vi "_builtins_resize_window.vi"(8 "error in (no error)":errorcluster, 10 "Focus":enum8{"FP", "BD"}(ring), 11 "VI Refnum in":refnum<vi>) -> (0 "error out":errorcluster, 3 "VI Refnum out":refnum<vi>)   [LabVIEW 2019, in "Script.lvlib"]
doc: "Resizes the front panel or block diagram window to content. On the front panel, this also resets the origins to 0, 0.\n\nCreated by: Ryan Pacini"
uses:
  Script.lvlib
  <vilib>/Utility/miscctls.llb/LVBoundsTypeDef.ctl
  <vilib>/Utility/miscctls.llb/LVPointTypeDef.ctl
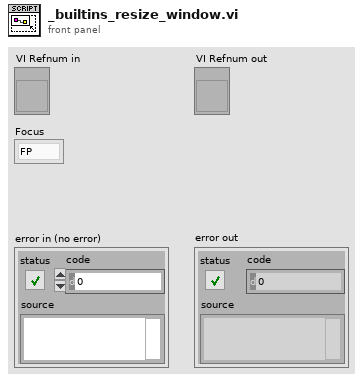
[diagram p1: front panel]
types:
  T1 = typedef "LVAllMonitorsDisplayTypeDef.ctl" = cluster{"Bounds":cluster{"Left":i16, "Top":i16, "Right":i16, "Bottom":i16}, "Depth":i16}[]
  T2 = typedef "LVBoundsTypeDef.ctl" = cluster{"Width":u32, "Height":u32}
  T3 = cluster{"Left":i16, "Top":i16, "Right":i16, "Bottom":i16}
  T4 = typedef "LVRectTypeDef.ctl" = cluster{"Left":i16, "Top":i16, "Right":i16, "Bottom":i16}
  T5 = typedef "LVPointTypeDef.ctl" = cluster{"Horizontal":i16, "Vertical":i16}
  T6 = typedef "LVPositionTypeDef.ctl" = cluster{"Left":i32, "Top":i32}
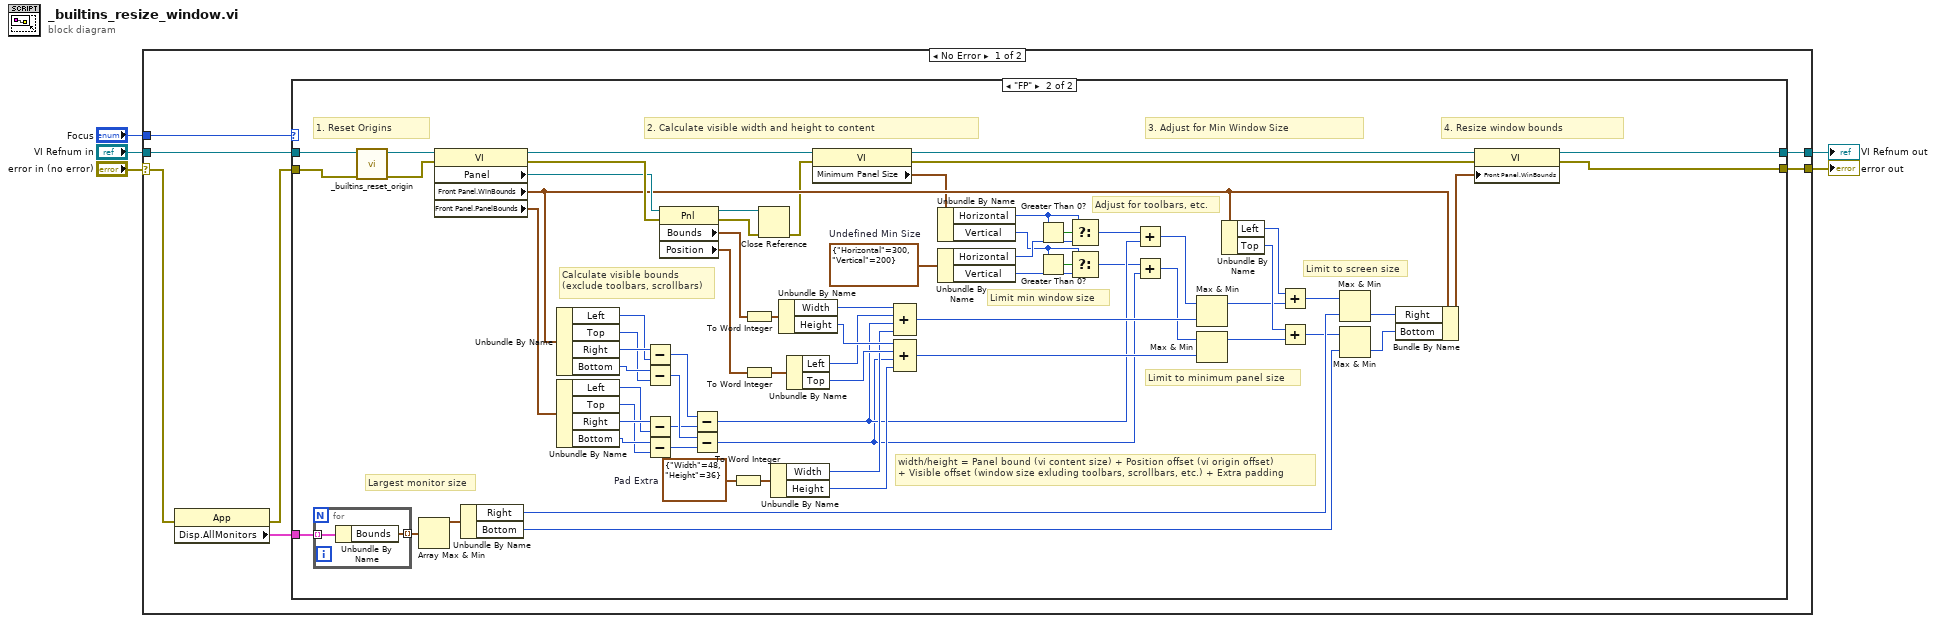
[diagram p0: block diagram]
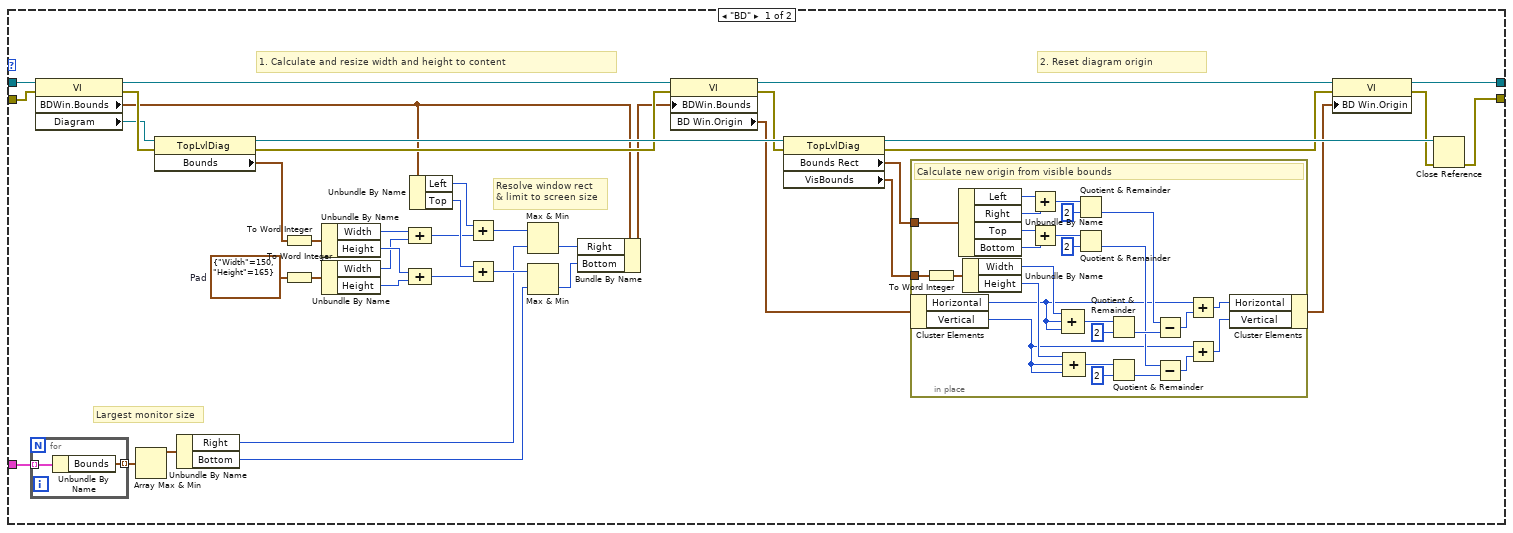
[diagram p2: hidden frame]
diagram:
  n1 = case shown="No Error" "error in (no error)" {
    selector: "error in (no error)" -> [w7 w155]
    tunnel: [w12 w156] -> w5
    tunnel: "VI Refnum in" -> [w11 w156]
    tunnel: [w10 w155] -> w2
    tunnel: "Focus" -> [w9 _]
    frame No Error {
      n2 = property class="App"(error in=w7) -> (error out=w6:errorcluster, "Disp.AllMonitors"=w8:T1)  [unwired: 1 in, 1 out]
      n3 = case shown="\"FP\"" w9 {
        tunnel: [w53 w152] -> w12
        tunnel: w11 -> [w52 w109]
        tunnel: w6 -> [w51 w111]
        tunnel: [w36 w107] -> w10
        tunnel: w8 -> [w14 w113]
        frame "BD" {
          w17 = T2 {"Width"=150, "Height"=165}  # Pad
          # "Largest monitor size"
          # "2. Reset diagram origin"
          # "1. Calculate and resize width and height to content"
          # "Resolve window rect\n& limit to screen size"
          n4 = for {
            tunnel: w14 -> [w82] mode=indexing
            tunnel: [w81] -> w37 mode=indexing
            n5 = Unbundle By Name(w82) -> ("Bounds"=w81:T3)
          }
          n6 = property on="Property Node" class="VI"(reference=w52, error in=w51) -> (reference out=w13:refnum<vi>, error out=w43:errorcluster, "BDWin.Bounds"=w25:T4, "Diagram"=w19:refnum<vi>)
          n7 = Array Max & Min(array=w37) -> (max value=w44:T3)  [unwired: 3 out]
          n8 = property on="Property Node" class="TopLvlDiag"(reference=w19, error in=w43) -> (reference out=w49:refnum<vi>, error out=w42:errorcluster, "Bounds"=w34:T2)
          n9 = Unbundle By Name(w44) -> ("Right"=w22:i16, "Bottom"=w21:i16)
          n10 = To Word Integer(number=w34) -> (16bit integer=w35:cluster{"Width":i16, "Height":i16})
          n11 = To Word Integer(number=w17) -> (16bit integer=w18:cluster{"Width":i16, "Height":i16})
          n12 = Unbundle By Name(w35) -> ("Width"=w32:i16, "Height"=w33:i16)
          n13 = Unbundle By Name(w18) -> ("Width"=w15:i16, "Height"=w16:i16)
          n14 = Compound Arithmetic op=ADD(w32, w15) -> (w24:i16)
          n15 = Compound Arithmetic op=ADD(w33, w16) -> (w23:i16)
          n16 = Unbundle By Name(w25) -> ("Left"=w29:i16, "Top"=w26:i16)
          n17 = Add(x=w29, y=w24) -> (x+y=w28:i16)
          n18 = Add(x=w26, y=w23) -> (x+y=w27:i16)
          n19 = Max & Min(x=w28, y=w22) -> (min(x,y)=w30:i16)  [unwired: 1 out]
          n20 = Max & Min(x=w27, y=w21) -> (min(x,y)=w31:i16)  [unwired: 1 out]
          n21 = Bundle By Name(cluster=w25, "Right"=w30, "Bottom"=w31) -> (w20:T4)
          n22 = property on="Property Node" class="VI"(reference=w13, error in=w42, "BDWin.Bounds"=w20) -> (reference out=w48:refnum<vi>, error out=w41:errorcluster, "BD Win.Origin"=w46:T5)
          n23 = property on="Property Node" class="TopLvlDiag"(reference=w49, error in=w41) -> (reference out=w50:refnum<vi>, error out=w39:errorcluster, "Bounds Rect"=w40:T4, "VisBounds"=w45:T2)
          n24 = in-place {
            in-place-border: w40 -> [w76]
            in-place-border: w45 -> [w64]
            # "Calculate new origin from visible bounds"
            n25 = in-place-cluster #1(w46) -> ("Horizontal"=w58:i16, "Vertical"=w57:i16)
            n26 = To Word Integer(number=w64) -> (16bit integer=w63:cluster{"Width":i16, "Height":i16})
            n27 = Unbundle By Name(w76) -> ("Left"=w80:i16, "Right"=w79:i16, "Top"=w78:i16, "Bottom"=w77:i16)
            n28 = Unbundle By Name(w63) -> ("Width"=w60:i16, "Height"=w62:i16)
            n29 = Add(x=w80, y=w79) -> (x+y=w75:i16)
            n30 = Add(x=w78, y=w77) -> (x+y=w74:i16)
            n31 = Compound Arithmetic op=ADD(w60, w58, w58) -> (w59:i16)
            n32 = Compound Arithmetic op=ADD(w62, w57, w57) -> (w61:i16)
            n33 = Quotient & Remainder(x=w75, y=i16 2) -> (floor(x/y)=w70:i16)  [unwired: 1 out]
            n34 = Quotient & Remainder(x=w74, y=i16 2) -> (floor(x/y)=w67:i16)  [unwired: 1 out]
            n35 = Quotient & Remainder(x=w59, y=i16 2) -> (floor(x/y)=w71:i16)  [unwired: 1 out]
            n36 = Quotient & Remainder(x=w61, y=i16 2) -> (floor(x/y)=w69:i16)  [unwired: 1 out]
            n37 = Subtract(x=w70, y=w71) -> (x-y=w66:i16)
            n38 = Subtract(x=w67, y=w69) -> (x-y=w65:i16)
            n39 = Add(x=w58, y=w66) -> (x+y=w56:i16)
            n40 = Add(x=w57, y=w65) -> (x+y=w55:i16)
            n41 = in-place-cluster #1("Horizontal"=w56, "Vertical"=w55) -> (w47:T5)
          }
          n42 = property on="Property Node" class="VI"(reference=w48, error in=w39, "BD Win.Origin"=w47) -> (reference out=w53:refnum<vi>, error out=w38:errorcluster)
          n43 = Close Reference(reference=w50, error in (no error)=w38) -> (error out=w36:errorcluster)
        }
        frame "FP" {
          w91 = T5 {"Horizontal"=300, "Vertical"=200}  # Undefined Min Size
          w116 = T2 {"Width"=48, "Height"=36}  # Pad Extra
          # "width/height = Panel bound (vi content size) + Position offset (vi origin offset)\n+ Visible offset (window size exluding toolbars, scrollbars, etc.) + Extra padding"
          # "4. Resize window bounds"
          # "3. Adjust for Min Window Size"
          # "Adjust for toolbars, etc."
          # "Limit min window size"
          # "Limit to minimum panel size"
          # "Largest monitor size"
          # "Calculate visible bounds\n(exclude toolbars, scrollbars)"
          # "1. Reset Origins"
          # "2. Calculate visible width and height to content"
          # "Limit to screen size"
          n44 = for {
            tunnel: w113 -> [w154] mode=indexing
            tunnel: [w153] -> w141 mode=indexing
            n45 = Unbundle By Name(w154) -> ("Bounds"=w153:T3)
          }
          n46 = call "_builtins_reset_origin.vi"("error in (no error)"=w111, "VI Refnum in"=w109) -> ("error out"=w112:errorcluster, "VI Refnum out"=w110:refnum<vi>)  [unwired: 8 in]
          n47 = Array Max & Min(array=w141) -> (max value=w150:T3)  [unwired: 3 out]
          n48 = property on="Property Node" class="VI"(reference=w110, error in=w112) -> (reference out=w104:refnum<vi>, error out=w147:errorcluster, "Panel"=w144:refnum<vi>, "Front Panel.WinBounds"=w130:T4, "Front Panel.PanelBounds"=w140:T4)
          n49 = Unbundle By Name(w150) -> ("Right"=w142:i16, "Bottom"=w143:i16)
          n50 = Unbundle By Name(w130) -> ("Left"=w125:i16, "Top"=w123:i16, "Right"=w127:i16, "Bottom"=w126:i16)
          n51 = Unbundle By Name(w140) -> ("Left"=w121:i16, "Top"=w119:i16, "Right"=w129:i16, "Bottom"=w128:i16)
          n52 = Subtract(x=w127, y=w125) -> (x-y=w124:i16)
          n53 = Subtract(x=w126, y=w123) -> (x-y=w122:i16)
          n54 = Subtract(x=w129, y=w121) -> (x-y=w120:i16)
          n55 = Subtract(x=w128, y=w119) -> (x-y=w118:i16)
          n56 = property on="Property Node" class="Pnl"(reference=w144, error in=w147) -> (reference out=w106:refnum<vi>, error out=w105:errorcluster, "Bounds"=w146:T2, "Position"=w108:T6)
          n57 = Subtract(x=w124, y=w120) -> (x-y=w95:i16)
          n58 = Subtract(x=w122, y=w118) -> (x-y=w92:i16)
          n59 = To Word Integer(number=w116) -> (16bit integer=w117:cluster{"Width":i16, "Height":i16})
          n60 = To Word Integer(number=w146) -> (16bit integer=w151:cluster{"Width":i16, "Height":i16})
          n61 = To Word Integer(number=w108) -> (16bit integer=w136:cluster{"Left":i16, "Top":i16})
          n62 = Close Reference(reference=w106, error in (no error)=w105) -> (error out=w102:errorcluster)
          n63 = Unbundle By Name(w117) -> ("Width"=w115:i16, "Height"=w114:i16)
          n64 = Unbundle By Name(w151) -> ("Width"=w139:i16, "Height"=w138:i16)
          n65 = Unbundle By Name(w136) -> ("Left"=w137:i16, "Top"=w135:i16)
          n66 = property class="VI"(reference=w104, error in=w102) -> (reference out=w103:refnum<vi>, error out=w101:errorcluster, "Minimum Panel Size"=w100:T5)
          n67 = Compound Arithmetic op=ADD(w139, w137, w95, w115) -> (w99:i16)
          n68 = Compound Arithmetic op=ADD(w138, w135, w92, w114) -> (w97:i16)
          n69 = Unbundle By Name(w100) -> ("Horizontal"=w89:i16, "Vertical"=w85:i16)
          n70 = Unbundle By Name(w91) -> ("Horizontal"=w87:i16, "Vertical"=w84:i16)
          n71 = Greater Than 0?(x=w89) -> (x > 0?=w90:bool)
          n72 = Greater Than 0?(x=w85) -> (x > 0?=w86:bool)
          n73 = Select(t=w89, s=w90, f=w87) -> (s? t:f=w88:i16)
          n74 = Select(t=w85, s=w86, f=w84) -> (s? t:f=w83:i16)
          n75 = Add(x=w88, y=w95) -> (x+y=w94:i16)
          n76 = Add(x=w83, y=w92) -> (x+y=w93:i16)
          n77 = Max & Min(x=w94, y=w99) -> (max(x,y)=w98:i16)  [unwired: 1 out]
          n78 = Max & Min(x=w93, y=w97) -> (max(x,y)=w96:i16)  [unwired: 1 out]
          n79 = Unbundle By Name(w130) -> ("Left"=w134:i16, "Top"=w131:i16)
          n80 = Add(x=w134, y=w98) -> (x+y=w133:i16)
          n81 = Add(x=w131, y=w96) -> (x+y=w132:i16)
          n82 = Max & Min(x=w133, y=w142) -> (min(x,y)=w148:i16)  [unwired: 1 out]
          n83 = Max & Min(x=w132, y=w143) -> (min(x,y)=w149:i16)  [unwired: 1 out]
          n84 = Bundle By Name(cluster=w130, "Right"=w148, "Bottom"=w149) -> (w145:T4)
          n85 = property on="Property Node" class="VI"(reference=w103, error in=w101, "Front Panel.WinBounds"=w145) -> (reference out=w152:refnum<vi>, error out=w107:errorcluster)
        }
      }
    }
    frame Error {
    }
  }
  "VI Refnum out" <- w5
  "error out" <- w2
